vi "MeasureOverlappedIV.vi"(7 "SMU":T1, 8 "Error In":errorcluster, 11 "Keithley 2602 In":refnum<visa-resource-name>) -> (0 "Error Out":errorcluster, 3 "Keithley 2602 Out":refnum<visa-resource-name>)   [LabVIEW 2012, in "Keithley-2602.lvlib"]
uses:
  Keithley-2602.lvlib
  Controls/SMU.ctl
panel:
  out "Command":string
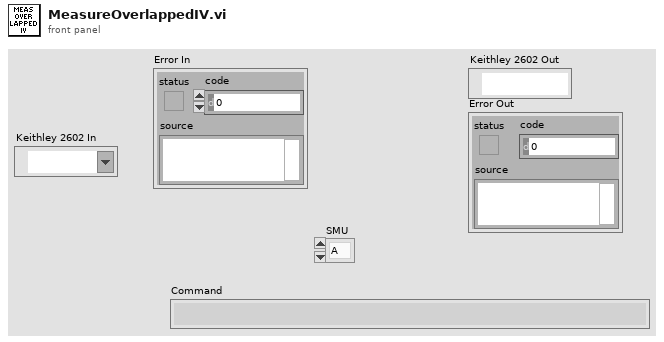
[diagram p1: front panel]
types:
  T1 = typedef "Keithley-2602.lvlib/SMU.ctl" = enum16{"A", "B"}
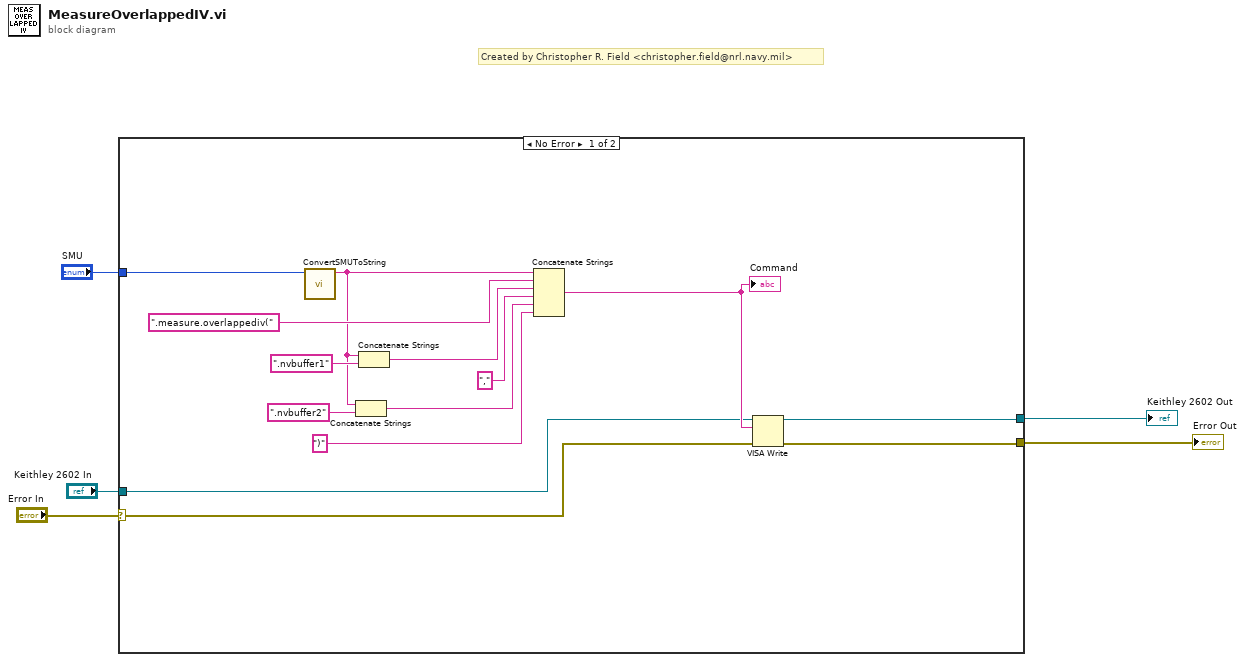
[diagram p0: block diagram]
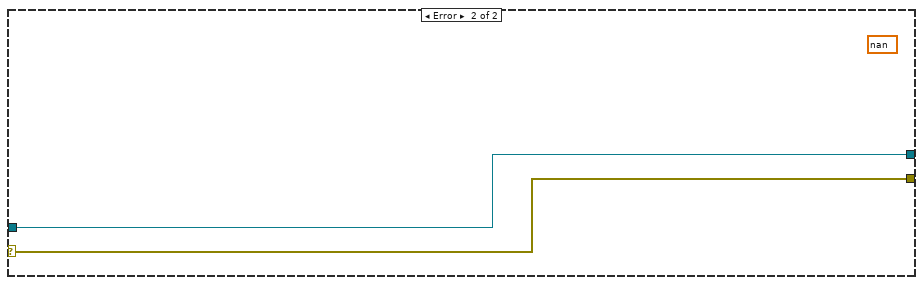
[diagram p2: hidden frame]
diagram:
  # "Created by Christopher R. Field <christopher.field@nrl.navy.mil>"
  n1 = case shown="No Error" "Error In" {
    selector: "Error In" -> [w15 w20]
    tunnel: [w7 w21] -> w5
    tunnel: [w6 w20] -> w4
    tunnel: "SMU" -> [w17 _]
    tunnel: "Keithley 2602 In" -> [w16 w21]
    frame No Error {
      n2 = call "ConvertSMUToString.vi"("SMU"=w17) -> ("Channel"=w13:string)  [unwired: 10 in]
      n3 = Concatenate Strings(w13, ".nvbuffer2" ("string")) -> (w9:string)
      n4 = Concatenate Strings(w13, ".nvbuffer1" ("string")) -> (w11:string)
      n5 = Concatenate Strings(w13, ".measure.overlappediv(", w11, "," ("string"), w9, ")" ("string")) -> (w18:string)
      "Command" <- w18
      n6 = VISA Write(VISA resource name=w16, write buffer=w18, error in (no error)=w15) -> (VISA resource name out=w7:refnum<visa-resource-name>, error out=w6:errorcluster)  [unwired: 1 out]
    }
    frame Error {
      (unwired) nan
    }
  }
  "Keithley 2602 Out" <- w5
  "Error Out" <- w4
